vi "LV SciSDK OSCILLOSCOPE RESET READ VALID FLAG.vi"(8 "error in (no error)":errorcluster, 9 "Oscilloscope Handle In":T1) -> (0 "error out":errorcluster, 1 "Oscilloscope Handle Out":T1)   [LabVIEW 2021]
uses:
  SciSDK_Labview.lvlib
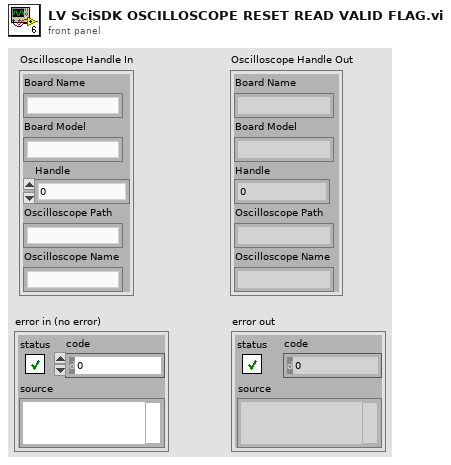
[diagram p1: front panel]
types:
  T1 = cluster{"Board Name":string, "Board Model":string, "Handle":u64, "Oscilloscope Path":string, "Oscilloscope Name":string}
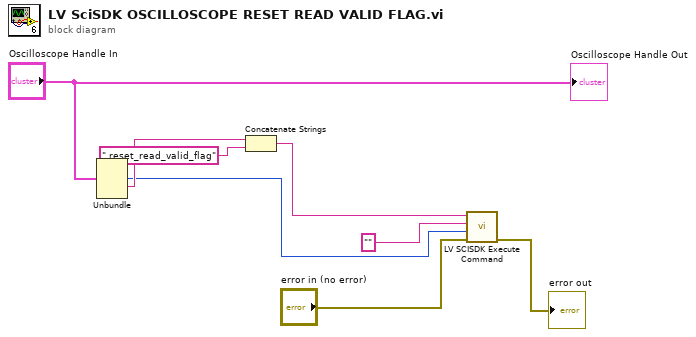
[diagram p0: block diagram]
diagram:
  n1 = Unbundle("Oscilloscope Handle In") -> ("Handle"=w3:u64, "Oscilloscope Path"=w7:string)  [unwired: 3 out]
  n2 = Concatenate Strings(w7, ".reset_read_valid_flag" ("string")) -> (w5:string)
  n3 = call "LV SCISDK Execute Command.vi"("error in (no error)"="error in (no error)", "handle"=w3, "value"="", "Path"=w5) -> ("error out"=→"error out":errorcluster)  [unwired: 5 in, 2 out]
  "Oscilloscope Handle Out" <- "Oscilloscope Handle In"
